vi "add scan temp(SubVI).vi"(6 "limit":T1, 10 "字符串":string) -> (0 "布尔 3":bool, 2 "连接的字符串":string)   [LabVIEW 2019, in "Add Seq.lvlib"]
uses:
  Add Seq.lvlib
  ctl/limit.ctl
  SubVI.lvlib
panel:
  in  "Number of Step":i32=10 min=0 max=70001
  in  "Step Delay(secs)":dbl
  in  "Approach":i32(ring)=2 items=["FastSettle", "NoOvershoot", "Sweep"]
  in  "Increments(K)":dbl=10.0
  in  "cancel":bool
  in  "ok":bool
  in  "Rate(K/min)":dbl=10.0 min=0.0 max=10.0
  in  "Final Temp(K)":dbl=300.0 min=2.0 max=325.0
  in  "Initial Temp(K)":dbl=300.0 min=2.0 max=325.0
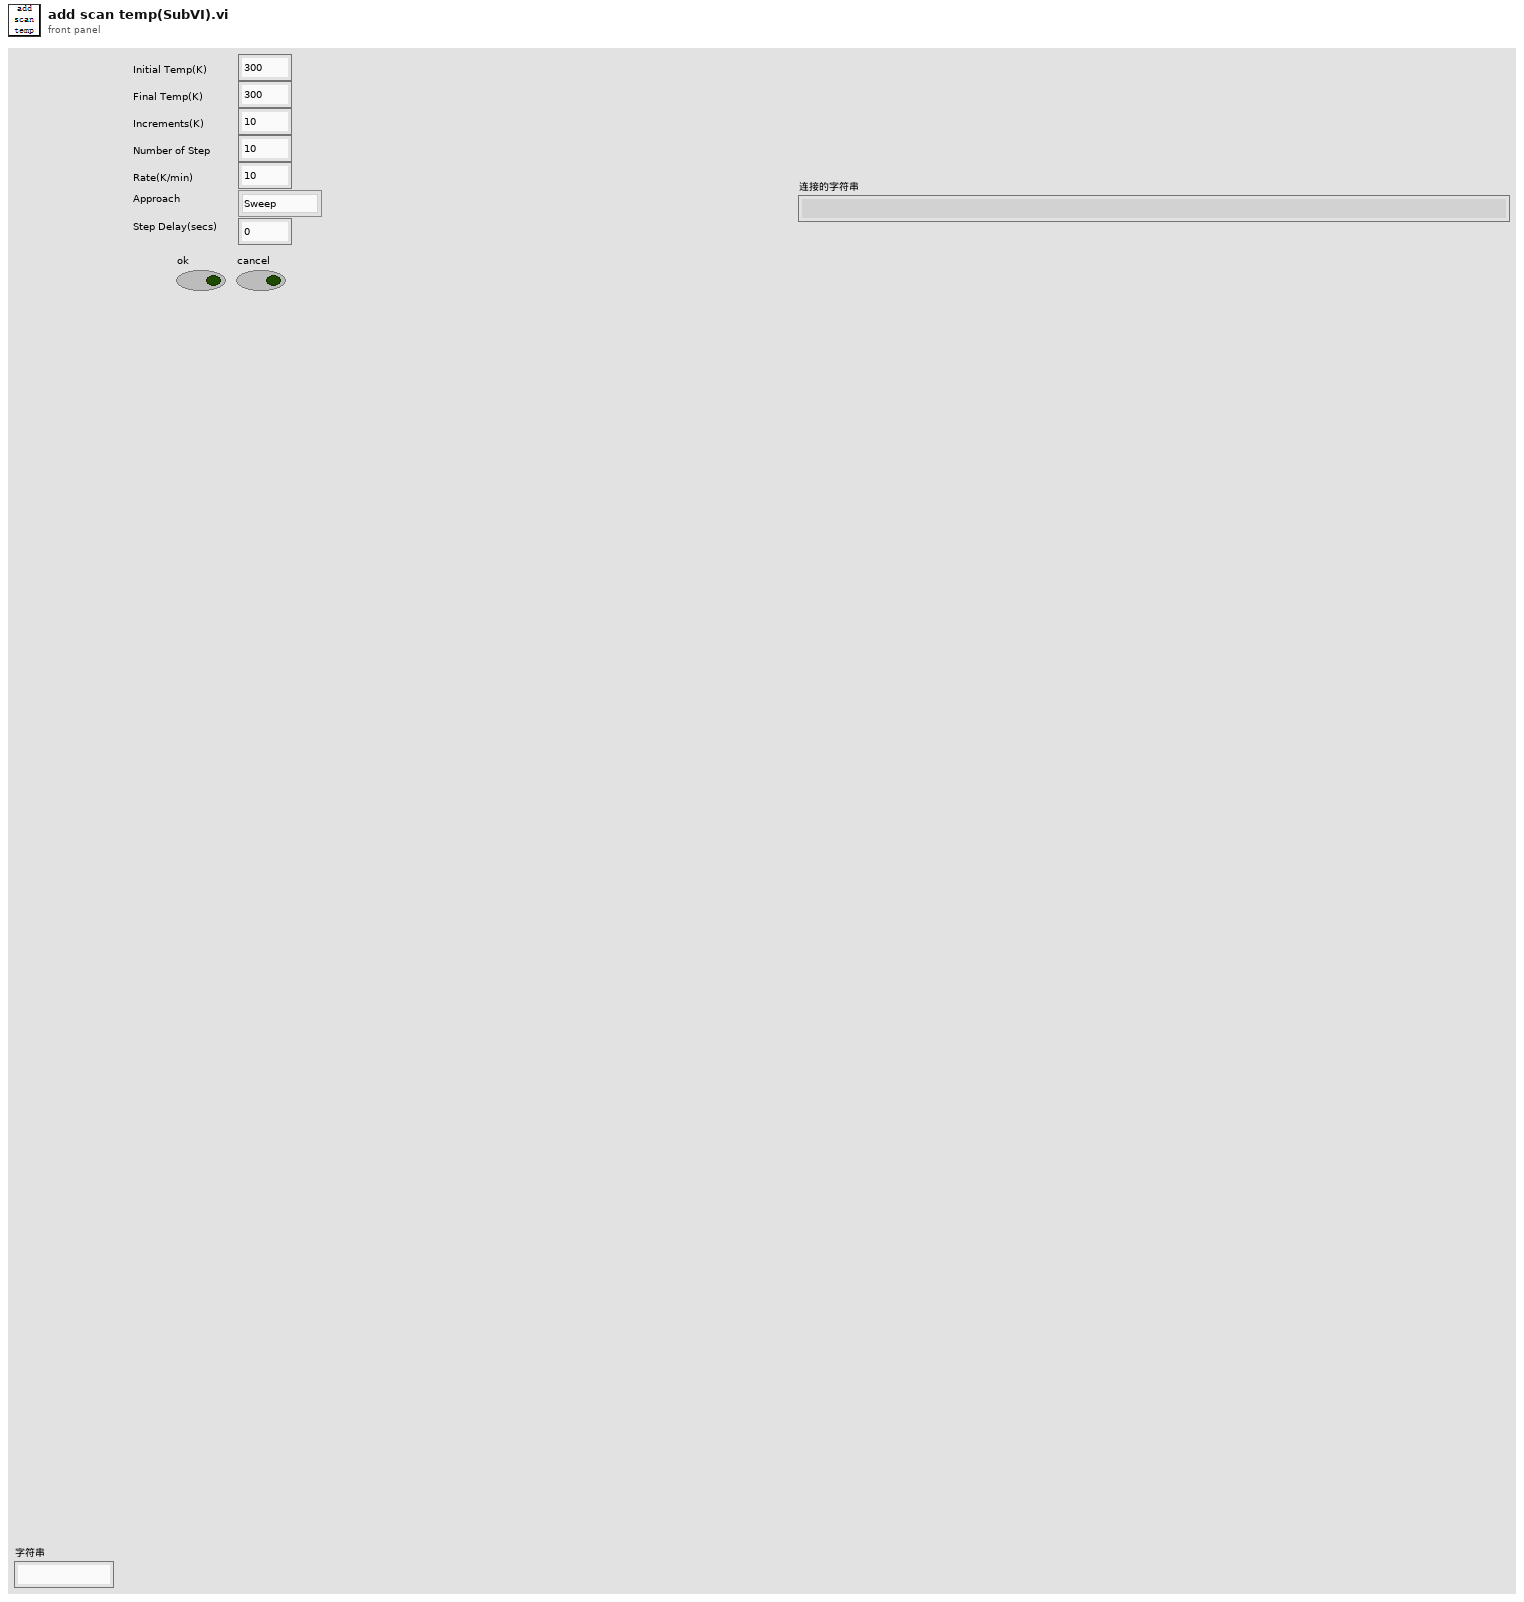
[diagram p1: front panel]
types:
  T1 = typedef "limit.ctl" = cluster{"Field limit":dbl, "Field rate limit":dbl, "Temp limit":dbl, "Temp low limit":dbl, "Temp rate limit ":dbl}
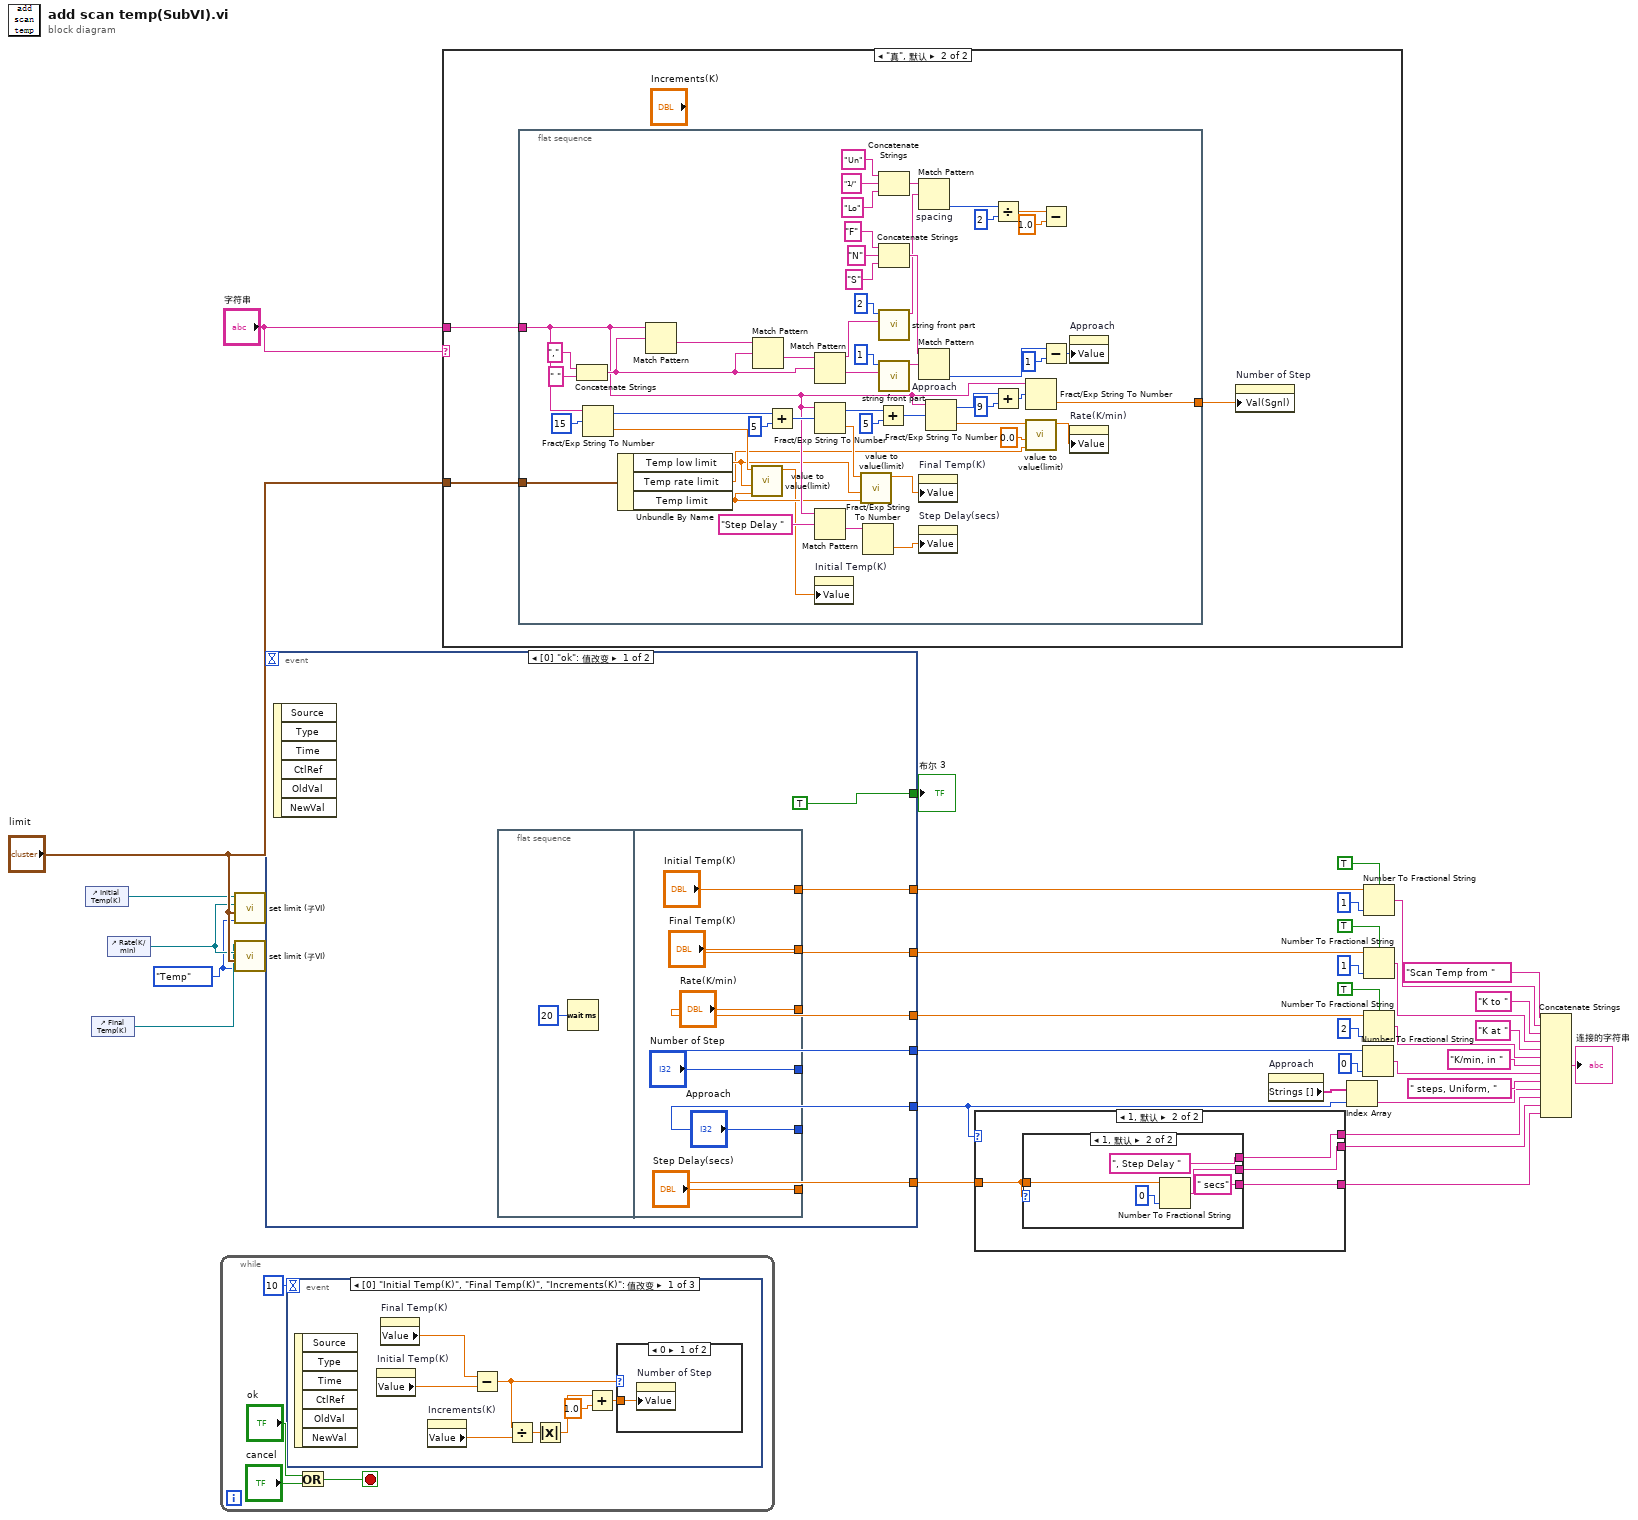
[diagram p0: block diagram]
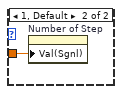
[diagram p3: hidden frame]
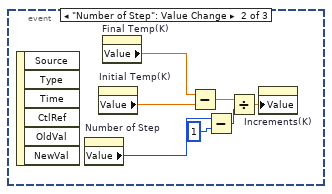
[diagram p4: hidden frame]
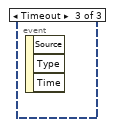
[diagram p5: hidden frame]
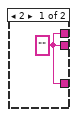
[diagram p6: hidden frame]
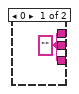
[diagram p7: hidden frame]
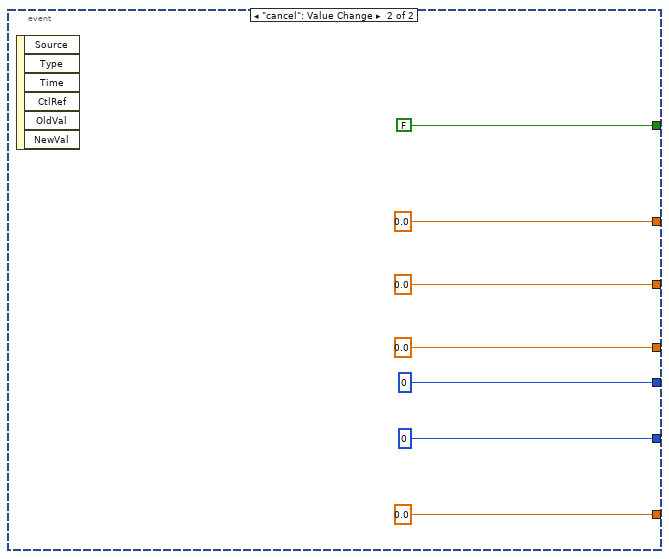
[diagram p8: hidden frame]
diagram:
  w1 = enum16{"Field", "Temp"}."Temp" ("Temp or Field")
  n1 = control-ref of="Initial Temp(K)"() -> (w2:refnum<vi>)
  n2 = control-ref of="Final Temp(K)"() -> (w3:refnum<vi>)
  n3 = control-ref of="Rate(K/min)"() -> (w4:refnum<vi>)
  n4 = while {
    stop <- w36 stop-if-true
    n5 = event shown="[0] \"Initial Temp(K)\", \"Final Temp(K)\", \"Increments(K)\": 值改变" {
      selector: _ -> [_ _ _]
      dyn-events: _ -> [_ _ _]
      timeout: 10 -> [_ _ _]
      event "Initial Temp(K)", "Final Temp(K)", "Increments(K)": Value Change {
        n6 = event-data() -> ()  [unwired: 1 in, 6 out]
        n7 = property on="Initial Temp(K)" class="DigNum (严格)"() -> ("Value"=w47:dbl)  [unwired: 2 in, 2 out]
        n8 = property on="Final Temp(K)" class="DigNum (严格)"() -> ("Value"=w42:dbl)  [unwired: 2 in, 2 out]
        n9 = property on="Increments(K)" class="DigNum (严格)"() -> ("Value"=w46:dbl)  [unwired: 2 in, 2 out]
        n10 = Subtract(x=w42, y=w47) -> (x-y=w41:dbl)
        n11 = Divide(x=w41, y=w46) -> (x/y=w44:dbl)
        n12 = Absolute Value(x=w44) -> (abs(x)=w43:dbl)
        n13 = Add(x=w43, y=1.0) -> (x+y=w40:dbl)
        n14 = case shown="0" w41 {
          tunnel: w40 -> [w48 w49]
          frame 0 {
            n15 = property on="Number of Step" class="DigNum (严格)"("Value"=w48) -> ()  [unwired: 2 in, 2 out]
          }
          frame 1, Default {
            n16 = property on="Number of Step" class="DigNum (严格)"("Val(Sgnl)"=w49) -> ()  [unwired: 2 in, 2 out]
          }
        }
      }
      event "Number of Step": Value Change {
        n17 = event-data() -> ()  [unwired: 1 in, 6 out]
        n18 = property on="Number of Step" class="DigNum (严格)"() -> ("Value"=w53:i32)  [unwired: 2 in, 2 out]
        n19 = property on="Initial Temp(K)" class="DigNum (严格)"() -> ("Value"=w55:dbl)  [unwired: 2 in, 2 out]
        n20 = property on="Final Temp(K)" class="DigNum (严格)"() -> ("Value"=w56:dbl)  [unwired: 2 in, 2 out]
        n21 = Subtract(x=w56, y=w55) -> (x-y=w54:dbl)
        n22 = Subtract(x=w53, y=1) -> (x-y=w51:i32)
        n23 = Divide(x=w54, y=w51) -> (x/y=w50:dbl)
        n24 = property on="Increments(K)" class="DigNum (严格)"("Value"=w50) -> ()  [unwired: 2 in, 2 out]
      }
      event Timeout {
        n25 = event-data() -> ()  [unwired: 1 in, 3 out]
      }
    }
    n26 = Or(x="ok", y="cancel") -> (x .or. y?=w36:bool)
  }
  n27 = call "set limit (子VI).vi"("Temp or Field"=w1, "limit"="limit", "rate"=w4, "value"=w2) -> ()  [unwired: 8 in]
  n28 = call "set limit (子VI).vi"("Temp or Field"=w1, "limit"="limit", "rate"=w4, "value"=w3) -> ()  [unwired: 8 in]
  n29 = event shown="[0] \"ok\": 值改变" {
    selector: _ -> [_ _]
    dyn-events: _ -> [_ _]
    timeout: _ -> [_ _]
    tunnel: [w63 0.0 ("Field 2")] -> w24
    tunnel: [w62 0.0 ("Rate输入")] -> w21
    tunnel: [w61 0.0 ("Field")] -> w33
    tunnel: [TRUE FALSE] -> w35
    tunnel: [w57 0 ("Number of Step")] -> w18
    tunnel: [w59 0 ("Approach输入")] -> w10
    tunnel: [w58 0.0 ("Step Delay(secs)")] -> w11
    event "ok": Value Change {
      n30 = event-data() -> ()  [unwired: 1 in, 6 out]
      n31 = flat-sequence {
        tunnel: ["Final Temp(K)"] -> w63
        tunnel: ["Rate(K/min)"] -> w62
        tunnel: ["Initial Temp(K)"] -> w61
        tunnel: ["Approach"] -> w59
        tunnel: ["Step Delay(secs)"] -> w58
        tunnel: ["Number of Step"] -> w57
        frame #0 {
          n32 = Wait (ms)(milliseconds to wait=u32 20 ("等待时间（毫秒）")) -> ()  [unwired: 1 out]
        }
        frame #1 {
        }
      }
    }
    event "cancel": Value Change {
      n33 = event-data() -> ()  [unwired: 1 in, 6 out]
    }
  }
  "布尔 3" <- w35
  n34 = case shown="\"真\", 默认" "字符串" {
    tunnel: "字符串" -> [_ w79]
    tunnel: "limit" -> [_ w78]
    frame "" {
    }
    frame "真", Default {
      n35 = flat-sequence {
        tunnel: [w97] -> w80
        tunnel: w79 -> [w92]
        tunnel: w78 -> [w91]
        frame #0 {
          n36 = Concatenate Strings("," ("字符串"), " " ("字符串")) -> (w114:string)
          n37 = Fract/Exp String To Number(string=w92, offset=15 ("偏移量")) -> (offset past number=w130:i32, number=w88:dbl)  [unwired: 2 in]
          n38 = Unbundle By Name(w91) -> ("Temp low limit"=w87:dbl, "Temp rate limit"=w84:dbl, "Temp limit"=w86:dbl)
          n39 = Match Pattern(string=w92, regular expression=w114) -> (after substring=w132:string)  [unwired: 1 in, 3 out]
          n40 = call "value to value(limit).vi"("high limit"=w86, "low limit"=w87, "数值 in"=w88) -> ("数值 out"=w85:dbl)  [unwired: 8 in]
          n41 = Match Pattern(string=w132, regular expression=w114) -> (after substring=w115:string)  [unwired: 1 in, 3 out]
          n42 = Add(x=w130, y=5) -> (x+y=w129:i32)
          n43 = Match Pattern(string=w115, regular expression=w114) -> (before substring=w113:string, after substring=w101:string)  [unwired: 1 in, 2 out]
          n44 = Fract/Exp String To Number(string=w92, offset=w129) -> (offset past number=w120:i32, number=w90:dbl)  [unwired: 2 in]
          n45 = Match Pattern(string=w92, regular expression="Step Delay ") -> (after substring=w99:string)  [unwired: 1 in, 3 out]
          n46 = property on="Initial Temp(K)" class="DigNum (严格)"("Value"=w85) -> ()  [unwired: 2 in, 2 out]
          n47 = call "value to value(limit).vi"("high limit"=w86, "low limit"=w87, "数值 in"=w90) -> ("数值 out"=w89:dbl)  [unwired: 8 in]
          n48 = Fract/Exp String To Number(string=w99) -> (number=w96:dbl)  [unwired: 3 in, 1 out]
          n49 = Add(x=w120, y=5) -> (x+y=w118:i32)
          n50 = Concatenate Strings("Un" ("字符串"), "1/" ("字符串"), "Lo" ("字符串")) -> (w107:string)
          n51 = Concatenate Strings("F" ("字符串"), "N" ("字符串"), "S" ("字符串")) -> (w123:string)
          n52 = call "string front part.vi"("字符串"=w113, "偏移量(0)"=2) -> ("result string"=w111:string)  [unwired: 9 in]
          n53 = call "string front part.vi"("字符串"=w101, "偏移量(0)"=1) -> ("result string"=w126:string)  [unwired: 9 in]
          n54 = Match Pattern "spacing"(string=w107, regular expression=w111) -> (offset past match=w106:i32)  [unwired: 1 in, 3 out]
          n55 = Match Pattern "Approach"(string=w123, regular expression=w126) -> (offset past match=w95:i32)  [unwired: 1 in, 3 out]
          n56 = property on="Final Temp(K)" class="DigNum (严格)"("Value"=w89) -> ()  [unwired: 2 in, 2 out]
          n57 = property on="Step Delay(secs)" class="DigNum (严格)"("Value"=w96) -> ()  [unwired: 2 in, 2 out]
          n58 = Fract/Exp String To Number(string=w92, offset=w118) -> (offset past number=w102:i32, number=w82:dbl)  [unwired: 2 in]
          n59 = Divide(x=w106, y=2) -> (x/y=w104:dbl)
          n60 = Add(x=w102, y=9) -> (x+y=w116:i32)
          n61 = Fract/Exp String To Number(string=w92, offset=w116) -> (number=w97:dbl)  [unwired: 2 in, 1 out]
          n62 = call "value to value(limit).vi"("high limit"=w84, "low limit"=0.0, "数值 in"=w82) -> ("数值 out"=w81:dbl)  [unwired: 8 in]
          n63 = Subtract(x=w104, y=1.0) -> ()  [unwired: 1 out]
          n64 = Subtract(x=w95, y=1) -> (x-y=w93:i32)
          n65 = property on="Approach" class="Ring (严格)"("Value"=w93) -> ()  [unwired: 2 in, 2 out]
          n66 = property on="Rate(K/min)" class="DigNum (严格)"("Value"=w81) -> ()  [unwired: 2 in, 2 out]
        }
      }
      n67 = property on="Number of Step" class="DigNum (严格)"("Val(Sgnl)"=w80) -> ()  [unwired: 2 in, 2 out]
    }
  }
  n68 = case shown="1, 默认" w10 {
    tunnel: [w133 w137] -> w9
    tunnel: [w133 w136] -> w7
    tunnel: w11 -> [_ w134]
    tunnel: [w133 w135] -> w8
    frame 2 {
      w133 = ""
    }
    frame 1, Default {
      n69 = case shown="1, 默认" w134 {
        tunnel: [w138 ", Step Delay " ("字符串")] -> w137
        tunnel: [w138 " secs" ("字符串")] -> w136
        tunnel: w134 -> [_ w141]
        tunnel: [w138 w140] -> w135
        frame 0 {
          w138 = ""
        }
        frame 1, Default {
          n70 = Number To Fractional String(number=w141, precision (6)=i16 0 ("精度(6)")) -> (F-format string=w140:string)  [unwired: 2 in]
        }
      }
    }
  }
  n71 = property on="Approach" class="Ring (严格)"() -> ("Strings []"=w12:string[])  [unwired: 2 in, 2 out]
  n72 = Index Array(array=w12, index=w10) -> (element=w14:string)
  n73 = Number To Fractional String(number=w18, precision (6)=i16 0 ("精度(6)")) -> (F-format string=w17:string)  [unwired: 2 in]
  n74 = Number To Fractional String(use system decimal point (T)=TRUE ("使用系统小数点(T)"), number=w33, precision (6)=i16 1 ("精度(6)")) -> (F-format string=w31:string)  [unwired: 1 in]
  n75 = Number To Fractional String(use system decimal point (T)=TRUE ("使用系统小数点(T)"), number=w24, precision (6)=i16 1 ("精度(6)")) -> (F-format string=w26:string)  [unwired: 1 in]
  n76 = Number To Fractional String(use system decimal point (T)=TRUE ("使用系统小数点(T)"), number=w21, precision (6)=i16 2 ("精度(6)")) -> (F-format string=w20:string)  [unwired: 1 in]
  n77 = Concatenate Strings("Scan Temp from " ("字符串"), w31, "K to " ("字符串"), w26, "K at " ("字符串"), w20, "K/min, in " ("字符串"), w17, " steps, Uniform, " ("字符串"), w14, w9, w8, w7) -> (→"连接的字符串":string)
